vi "Json Validate.vi"(6 "GenError(T)":bool=TRUE, 8 "error in (no error)":errorcluster, 11 "String":string) -> (0 "error out":errorcluster, 2 "Valid Json?":bool, 3 "Json without comments":string, 5 "String (dup)":string)   [LabVIEW 2019, in "lv-apt-json-file.lvlib"]
uses:
  lv-apt-json-file.lvlib
  <vilib>/Utility/error.llb/Error Cluster From Error Code.vi
  <vilib>/ErrorRing/Error Ring.xnode
  <vilib>/addons/_JKI.lib/Serialization/JSON/JKI JSON Serialization.lvlib
  <vilib>/JDP Science/JSONtext/JSONtext.lvlib
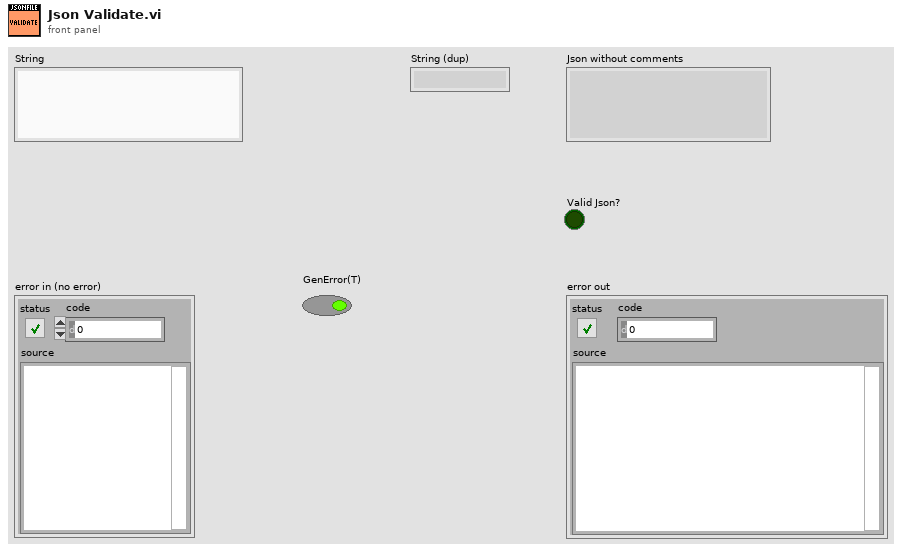
[diagram p1: front panel]
types:
  T1 = typedef "JSONtext.lvlib/JSON Value Type.ctl" = enum16{"Not a JSON Value", "JSON Object", "JSON Array", "String", "Number", "true", "false", "null"}
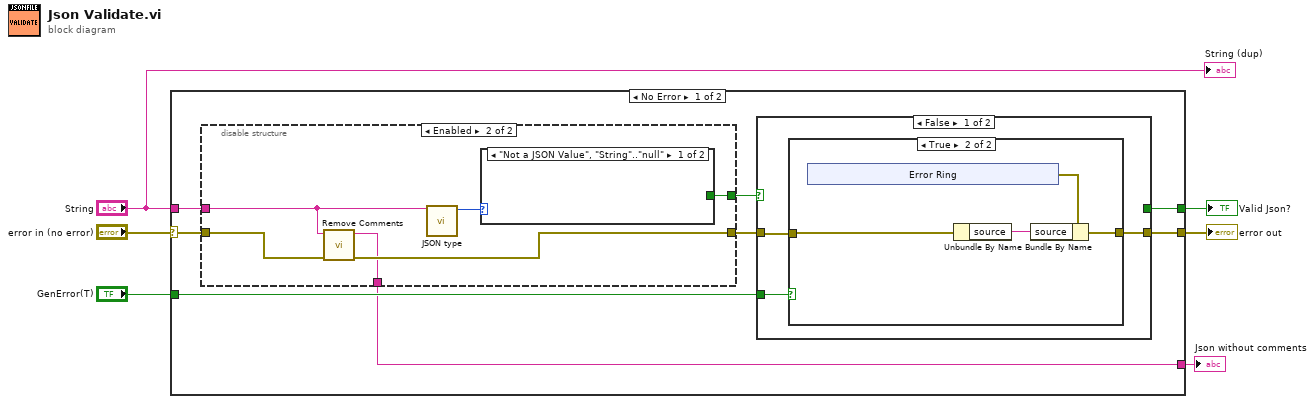
[diagram p0: block diagram]
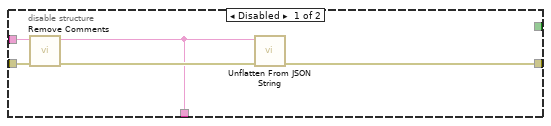
[diagram p2: hidden frame]
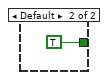
[diagram p3: hidden frame]
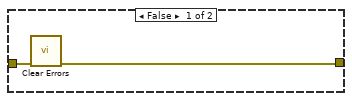
[diagram p4: hidden frame]
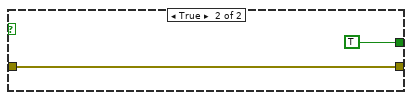
[diagram p5: hidden frame]
diagram:
  n1 = case shown="No Error" "error in (no error)" {
    selector: "error in (no error)" -> [w9 w42]
    tunnel: "String" -> [w10 _]
    tunnel: [w13 _] -> w5
    tunnel: [w12 w42] -> w4
    tunnel: "GenError(T)" -> [w11 _]
    tunnel: [w8 _] -> w1
    frame No Error {
      n2 = disable-structure shown="Enabled" {
        disable-tunnel: [w19 w21] -> w14
        disable-tunnel: w10 -> [w18 w23]
        disable-tunnel: w9 -> [w17 w22]
        disable-tunnel: [w15 w20] -> w8
        disable-tunnel: [_ w24] -> w7
        frame Disabled {
          n3 = call "Remove Comments.vi"("error in (no error)"=w17, "String"=w18) -> ("error out"=w16:errorcluster, "string"=w15:string)  [unwired: 8 in]
          n4 = call <vilib>:"Unflatten From JSON String.vi"("error in (no error)"=w16, "JSON String"=w15) -> ("error out"=w19:errorcluster)  [unwired: 8 in, 1 out]
        }
        frame Enabled {
          n5 = call "Remove Comments.vi"("error in (no error)"=w22, "String"=w23) -> ("error out"=w21:errorcluster, "string"=w20:string)  [unwired: 8 in]
          n6 = call <vilib>:"JSON type.vi"("JSON"=w23) -> ("JSON Value Type"=w25:T1)  [unwired: 9 in, 1 out]
          n7 = case shown="\"Not a JSON Value\", \"String\"..\"null\"" w25 {
            tunnel: [_ TRUE] -> w24
            frame "Not a JSON Value", "String".."null" {
            }
            frame Default {
            }
          }
        }
      }
      n8 = case shown="False" w7 {
        tunnel: [_ TRUE] -> w13
        tunnel: [w29 w40] -> w12
        tunnel: w11 -> [w27 _]
        tunnel: w14 -> [w28 w40]
        frame False {
          n9 = case shown="True" w27 {
            tunnel: [w30 w34] -> w29
            tunnel: w28 -> [w31 w33]
            frame False {
              n10 = call <vilib>:"Clear Errors.vi"("error in (no error)"=w31) -> ("error out"=w30:errorcluster)  [unwired: 5 in, 1 out]
            }
            frame True {
              n11 = xnode "Error Ring"() -> ("error out"=w35:errorcluster)
              n12 = Unbundle By Name(w33) -> ("source"=w32:string)
              n13 = Bundle By Name(cluster=w35, "source"=w32) -> (w34:errorcluster)
            }
          }
        }
        frame True {
        }
      }
    }
    frame Error {
    }
  }
  "error out" <- w4
  "Valid Json?" <- w5
  "Json without comments" <- w1
  "String (dup)" <- "String"
